vi "Sound Input to File.vi"() -> ()   [LabVIEW 2023]
doc: "This VI illustrates how to create a sound file using microphone input as data. It displays the sound data in a graph as it is written to the file."
uses:
  <vilib>/sound2/lvsound2.llb/Sampling Mode.ctl
  <vilib>/sound2/lvsound2.llb/Sound Data Format.ctl
  <vilib>/sound2/lvsound2.llb/Sound File Write Open.vi
  <vilib>/sound2/lvsound2.llb/Sound Input Read (DBL).vi
  <vilib>/sound2/lvsound2.llb/Sound File Write (DBL).vi
panel:
  out "Generated Sound File":path
  out "Waveform Graph":waveform(dbl)[](graph)
  in  "Stop":bool
  in  "Device ID":u32
  # "Overview: Demonstrates the use of the Sound Functions to create a sound file using microphone input as data.\nRequirements: Microphone\nInstructions:\n1. Specify the Device ID.\n2. Run the VI. The graph will show the data that is written to the sound file.\n3. Click Stop to stop the VI.\n4. Delete the generated sound file when you are done."
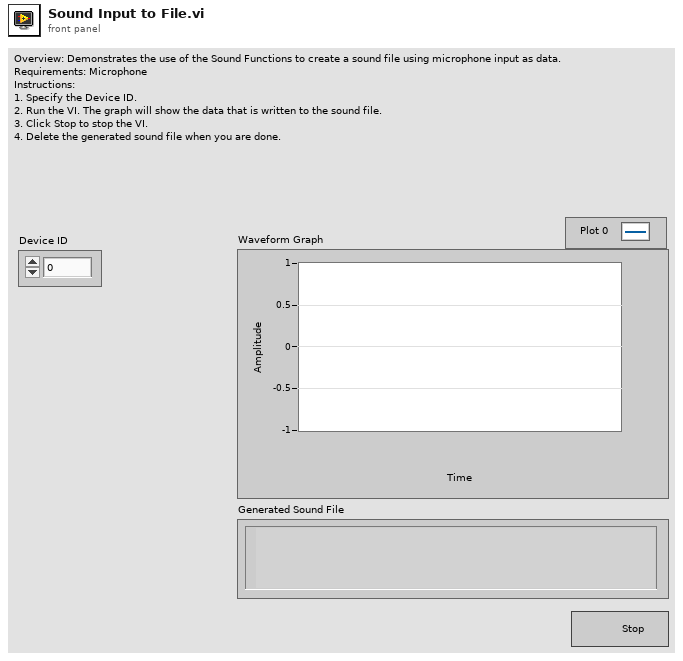
[diagram p1: front panel]
types:
  T1 = typedef "Sound Data Format.ctl" = cluster{"sample rate (S/s)":dbl, "number of channels":i32, "bits per sample":i32}
  T2 = typedef "Sampling Mode.ctl" = i32
  T3 = typedef "Sound File Refnum.ctl" = refnum<file>
  T4 = typedef "Sound Input Task ID.ctl" = u32
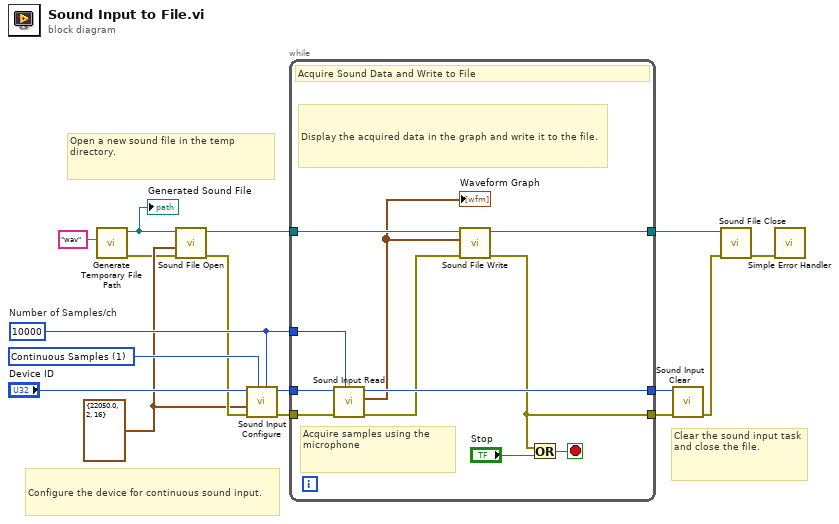
[diagram p0: block diagram]
diagram:
  w4 = T1 {"sample rate (S/s)"=22050.0, "number of channels"=2, "bits per sample"=16} ("Sound Format")
  w11 = 10000  # Number of Samples/ch
  w10 = T2 1 items=["Finite Samples", "Continuous Samples"] ("sample mode")
  # "Configure the device for continuous sound input."
  # "Clear the sound input task and close the file."
  # "Open a new sound file in the temp directory."
  n1 = call <vilib>:"Generate Temporary File Path.vi"("Temporary File Extension (tmp)"="wav") -> ("error out"=w3:errorcluster, "Unique Temporary File Path"=w1:path)  [unwired: 9 in]
  "Generated Sound File" <- w1
  n2 = call-poly <vilib>:"Sound File Open.vi"("error in (no error)"=w3, "sound format"=w4, "path"=w1) -> ("error out"=w6:errorcluster, "sound file refnum"=w9:T3)  [unwired: 7 in]
  n3 = call <vilib>:"Sound Input Configure.vi"("number of samples/ch"=w11, "sample mode"=w10, "error in (no error)"=w6, "sound format"=w4, "device ID"="Device ID") -> ("error out"=w16:errorcluster, "task ID"=w14:T4)  [unwired: 5 in]
  n4 = while {
    tunnel: w11 -> [w24]
    tunnel: w9 -> [w21]
    tunnel: [w20] -> w8
    tunnel: w14 -> [w26]
    tunnel: [w25] -> w13
    tunnel: w16 -> [w27]
    tunnel: [w17] -> w12
    stop <- w22 stop-if-true
    # "Acquire samples using the microphone"
    # "Display the acquired data in the graph and write it to the file."
    # "Acquire Sound Data and Write to File"
    n5 = call-poly <vilib>:"Sound Input Read.vi"("number of samples/ch"=w24, "error in (no error)"=w27, "task ID"=w26) -> ("error out"=w19:errorcluster, "data"=w18:waveform(dbl)[], "task ID out"=w25:T4)  [unwired: 6 in]
    "Waveform Graph" <- w18
    n6 = call-poly <vilib>:"Sound File Write.vi"("error in (no error)"=w19, "data"=w18, "sound file refnum"=w21) -> ("error out"=w17:errorcluster, "sound file refnum out"=w20:T3)  [unwired: 7 in]
    n7 = Or(x=w17, y="Stop") -> (x .or. y?=w22:bool)
  }
  n8 = call <vilib>:"Sound Input Clear.vi"("error in (no error)"=w12, "task ID"=w13) -> ("error out"=w7:errorcluster)  [unwired: 9 in]
  n9 = call <vilib>:"Sound File Close.vi"("error in (no error)"=w7, "sound file refnum"=w8) -> ("error out"=w5:errorcluster)  [unwired: 9 in]
  n10 = call <vilib>:"Simple Error Handler.vi"("error in (no error)"=w5) -> ()  [unwired: 4 in, 5 out]
